vi "DataAcquisition2.vi"() -> ()   [LabVIEW 2012]
panel:
  out "Waveform Graph":dynamicdata(graph)
  out "Array":dbl[](array[numeric])
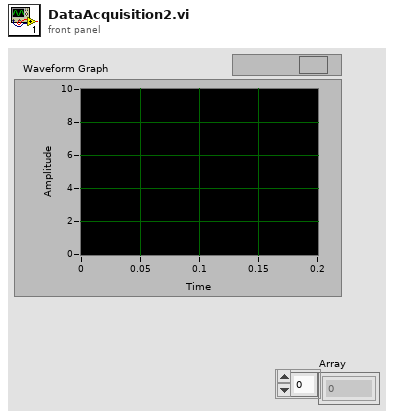
[diagram p1: front panel]
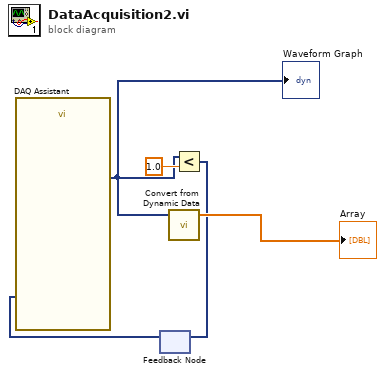
[diagram p0: block diagram]
diagram:
  n1 = feedback #1() -> (w1:dynamicdata)  [unwired: 1 in]
  n2 = call "DAQ Assistant"("stop (T)"=w1) -> ("data"=w3:dynamicdata)  [unwired: 16 in, 2 out]
  "Waveform Graph" <- w3
  n3 = call "Convert from Dynamic Data"("Dynamic Data Type"=w3) -> ("Array"=→"Array":dbl[])  [unwired: 3 in]
  n4 = Less?(x=w3, y=1.0) -> (x < y?=w2:dynamicdata)
  n5 = feedback-in #1(w2) -> ()
